vi "Lab Panel V4.84.vi"() -> ()   [LabVIEW 2013] (continued)
            n212 = case shown="True" w255 {
              frame False {
                n213 = local write "Message"("") -> ()
              }
              frame True {
                "Message" <- "NETWORK DIRECTORY NOT FOUND!!!!"
              }
            }
            n214 = property on="Message" class="Str"("Text.TextColor"=u32 16711680) -> ()  [unwired: 2 in, 2 out]
            n215 = property on="Network Directory" class="Path"("Blinking"=w253) -> ()  [unwired: 2 in, 2 out]
            n216 = property on="Message" class="Str"("Blinking"=w253) -> ()  [unwired: 2 in, 2 out]
          }
        }
        frame #10 {
          w261 = FALSE
          n217 = property on="Message" class="Str"("Blinking"=w261) -> ()  [unwired: 2 in, 2 out]
          n218 = property on="Network Directory" class="Path"("Blinking"=w261) -> ()  [unwired: 2 in, 2 out]
          n219 = property on="Tab Control 2" class="TabCtl (strict)"("Value"=0) -> ()  [unwired: 2 in, 2 out]
        }
      }
    }
    frame #2 {
      n220 = node-c288("loop  delay(mS)") -> (w265:T15)  [unwired: 3 in]
      n221 = timed-loop {
        timing: w265 -> [_]
        timing-out: [_] -> w264
        i -> [w287]
        stop <- "stop" stop-if-true
        n222 = node-c288() -> ()  [unwired: 1 in, 1 out]
        n223 = global write "Global display 1.vi" "stop disp"("stop") -> ()
        n224 = local read "SELECT LAB05-2"() -> (w267:T3)
        n225 = local read "SELECT LAB05-1"() -> (w268:T3)
        n226 = local read "SELECT LAB04-2"() -> (w269:T3)
        n227 = local read "SELECT LAB03-1"() -> (w272:T3)
        n228 = local read "SELECT LAB02-2"() -> (w273:T3)
        n229 = local read "SELECT LAB03-2"() -> (w271:T3)
        n230 = local read "SELECT LAB04-1"() -> (w270:T3)
        n231 = local read "SELECT LAB02-1"() -> (w274:T3)
        n232 = local read "TEST LAB01-1"() -> (w276:u16)
        n233 = local read "TEST LAB01-2"() -> (w275:T3)
        n234 = local read "run lab03-2"() -> (w281:bool)
        n235 = local read "run lab04-1"() -> (w280:bool)
        n236 = local read "run lab05-1"() -> (w278:bool)
        n237 = local read "run lab04-2"() -> (w279:bool)
        n238 = local read "run lab05-2"() -> (w277:bool)
        n239 = local read "run lab03-1"() -> (w282:bool)
        n240 = local read "run lab02-2"() -> (w283:bool)
        n241 = local read "run lab02-1"() -> (w284:bool)
        n242 = local read "run lab01-1"() -> (w286:bool)
        n243 = local read "run lab01-2"() -> (w285:bool)
        n244 = stacked-sequence {
          seq-local: [_ w349 _ _ _ _ _ _ _ _ _ _ _ _ _ _ _ _ _ _ _ _] -> [_ _ _ _ _ w2141 _ _ _ _ _ _ _ _ _ _ _ _ _ _ _ _]
          seq-local: [_ w348 _ _ _ _ _ _ _ _ _ _ _ _ _ _ _ _ _ _ _ _] -> [_ _ _ _ _ w2140 _ _ _ _ _ _ _ _ _ _ _ _ _ _ _ _]
          seq-local: [_ w335 _ _ _ _ _ _ _ _ _ _ _ _ _ _ _ _ _ _ _ _] -> [_ _ _ _ _ w2139 _ _ _ _ _ _ _ _ _ _ _ _ _ _ _ _]
          seq-local: [_ w334 _ _ _ _ _ _ _ _ _ _ _ _ _ _ _ _ _ _ _ _] -> [_ _ _ _ _ w2138 _ _ _ _ _ _ _ _ _ _ _ _ _ _ _ _]
          seq-local: [_ w333 _ _ _ _ _ _ _ _ _ _ _ _ _ _ _ _ _ _ _ _] -> [_ _ _ _ _ w2137 _ _ _ _ _ _ _ _ _ _ _ _ _ _ _ _]
          seq-local: [_ w332 _ _ _ _ _ _ _ _ _ _ _ _ _ _ _ _ _ _ _ _] -> [_ _ _ _ _ w2136 _ _ _ _ _ _ _ _ _ _ _ _ _ _ _ _]
          seq-local: [_ w331 _ _ _ _ _ _ _ _ _ _ _ _ _ _ _ _ _ _ _ _] -> [_ _ _ _ _ w2135 _ _ _ _ _ _ _ _ _ _ _ _ _ _ _ _]
          seq-local: [_ w330 _ _ _ _ _ _ _ _ _ _ _ _ _ _ _ _ _ _ _ _] -> [_ _ _ _ _ w2134 _ _ _ _ _ _ _ _ _ _ _ _ _ _ _ _]
          seq-local: [_ w329 _ _ _ _ _ _ _ _ _ _ _ _ _ _ _ _ _ _ _ _] -> [_ _ _ _ _ w2133 _ _ _ _ _ _ _ _ _ _ _ _ _ _ _ _]
          seq-local: [_ w328 _ _ _ _ _ _ _ _ _ _ _ _ _ _ _ _ _ _ _ _] -> [_ _ _ _ _ w2132 _ _ _ _ _ _ _ _ _ _ _ _ _ _ _ _]
          tunnel: w286 -> [_ _ w365 w607 w1731 w2161 w2471 w2718 _ _ _ _ w3122 _ w4056 _ _ w4339 w4642 w4824 _ _]
          tunnel: w285 -> [_ _ w364 w605 w1730 w2160 w2472 w2717 _ _ _ _ w3121 _ w4054 _ _ w4338 w4641 w4822 _ _]
          tunnel: w284 -> [_ _ w363 w603 w1729 w2159 w2470 w2716 _ _ _ _ w3120 _ w4052 _ _ w4337 w4640 w4821 _ _]
          tunnel: w283 -> [_ _ w362 w601 w1728 w2158 w2469 w2715 _ _ _ _ w3119 _ w4050 _ _ w4336 w4639 w4820 _ _]
          tunnel: w282 -> [_ _ w361 w599 w1727 w2157 w2468 w2714 _ _ _ _ w3118 _ w4048 _ _ w4335 w4638 w4819 _ _]
          tunnel: w281 -> [_ _ w360 w597 w1726 w2156 w2467 w2713 _ _ _ _ w3117 _ w4046 _ _ w4334 w4637 w4818 _ _]
          tunnel: w280 -> [_ _ w359 w595 w1725 w2155 w2466 w2712 _ _ _ _ w3116 _ w4044 _ _ w4333 w4636 w4817 _ _]
          tunnel: w279 -> [_ _ w358 w593 w1724 w2154 w2465 w2711 _ _ _ _ w3115 _ w4042 _ _ w4332 w4635 w4816 _ _]
          tunnel: w278 -> [_ _ w357 w591 w1723 w2153 w2464 w2710 _ _ _ _ w3114 _ w4040 _ _ w4331 w4634 w4815 _ _]
          tunnel: w277 -> [_ _ w356 w589 w1722 w2152 w2463 w2709 _ _ _ _ w3113 _ w4038 _ _ w4330 w4633 w4814 _ _]
          tunnel: w276 -> [_ _ _ w606 w1721 w2151 _ _ _ _ _ _ _ _ w4058 _ _ _ _ _ w5168 _]
          tunnel: w275 -> [_ _ _ w604 w1720 w2150 _ _ _ _ _ _ _ _ w4053 _ _ _ _ _ w5167 _]
          tunnel: w274 -> [_ _ _ w602 w1719 w2149 _ _ _ _ _ _ _ _ w4051 _ _ _ _ _ w5166 _]
          tunnel: w273 -> [_ _ _ w600 w1718 w2148 _ _ _ _ _ _ _ _ w4049 _ _ _ _ _ w5165 _]
          tunnel: w272 -> [_ _ _ w598 w1717 w2147 _ _ _ _ _ _ _ _ w4047 _ _ _ _ _ w5164 _]
          tunnel: w271 -> [_ _ _ w596 w1716 w2146 _ _ _ _ _ _ _ _ w4045 _ _ _ _ _ w5163 _]
          tunnel: w270 -> [_ _ _ w594 w1715 w2145 _ _ _ _ _ _ _ _ w4043 _ _ _ _ _ w5162 _]
          tunnel: w269 -> [_ _ _ w592 w1714 w2144 _ _ _ _ _ _ _ _ w4041 _ _ _ _ _ w5161 _]
          tunnel: w268 -> [_ _ _ w590 w1713 w2143 _ _ _ _ _ _ _ _ w4039 _ _ _ _ _ w5160 _]
          tunnel: w267 -> [_ _ _ w588 w1712 w2142 _ _ _ _ _ _ _ _ w4037 _ _ _ _ _ w5159 _]
          frame #0 {
            w291 = FALSE
            w296 = 0.5
            # "set up cycle control"
            n245 = local read "jig cycle"() -> (w295:dbl)
            n246 = Divide(x="JIG ON TIME (S)", y=w296) -> (x/y=→"on loops":dbl)
            n247 = Divide(x="JIG OFF TIME (S)", y=w296) -> (x/y=→"off loops":dbl)
            n248 = Increment(x=w295) -> (x+1=w294:dbl)
            n249 = local write "TEMP"(w291) -> ()
            n250 = local write "AI"(w291) -> ()
            n251 = local write "jig cycle"(w294) -> ()
            n252 = event shown="[1] \"ADMIN\": Value Change" {
              selector: _ -> [_ _]
              dyn-events: _ -> [_ _]
              timeout: 10 -> [_ _]
              event Timeout {
                n253 = event-data() -> ()  [unwired: 1 in, 3 out]
              }
              event "ADMIN": Value Change {
                n254 = event-data() -> ()  [unwired: 1 in, 6 out]
                n255 = stacked-sequence {
                  seq-local: [_ w300 _] -> [_ _ w301]
                  frame #0 {
                    n256 = global write "Global 1.vi" "password"("9999") -> ()
                  }
                  frame #1 {
                    n257 = call "sub vi - password 1.vi"() -> ("RESULT"=w300:bool)  [unwired: 11 in]
                  }
                  frame #2 {
                    w303 = FALSE
                    n258 = property on="Tab Control 2" class="TabCtl (strict)"() -> ("Pages"=w307:refnum<vi>[])  [unwired: 2 in, 2 out]
                    n259 = Select(t=TRUE, s=w301, f=w303) -> (s? t:f=w302:bool)
                    n260 = Index Array(array=w307, index=9) -> (element=w305:refnum<vi>)
                    n261 = property class="Page"(reference=w305, "PageVis"=w302) -> ()  [unwired: 1 in, 2 out]
                    n262 = local write "ADMIN"(w303) -> ()
                  }
                }
              }
            }
          }
          frame #1 {
            w345 = 60.0
            # "convert temperature rise minutes to cycles"
            n263 = local read "SET LAB05-2"() -> (w309:T5)
            n264 = local read "SET LAB05-1"() -> (w311:T5)
            n265 = local read "SET LAB04-2"() -> (w313:T5)
            n266 = local read "SET LAB01-1"() -> (w327:T5)
            n267 = local read "SET LAB01-2"() -> (w325:T5)
            n268 = local read "SET LAB02-2"() -> (w321:T5)
            n269 = local read "SET LAB04-1"() -> (w315:T5)
            n270 = local read "SET LAB03-1"() -> (w319:T5)
            n271 = local read "SET LAB03-2"() -> (w317:T5)
            n272 = local read "SET LAB02-1"() -> (w323:T5)
            n273 = local read "JIG OFF TIME (S)"() -> (w350:dbl)
            n274 = local read "JIG ON TIME (S)"() -> (w351:dbl)
            n275 = Unbundle(w309) -> ("T-RISE mins"=w308:dbl)  [unwired: 4 out]
            n276 = Unbundle(w311) -> ("T-RISE mins"=w310:dbl)  [unwired: 4 out]
            n277 = Unbundle(w327) -> ("T-RISE mins"=w326:dbl)  [unwired: 4 out]
            n278 = Unbundle(w313) -> ("T-RISE mins"=w312:dbl)  [unwired: 4 out]
            n279 = Unbundle(w325) -> ("T-RISE mins"=w324:dbl)  [unwired: 4 out]
            n280 = Unbundle(w323) -> ("T-RISE mins"=w322:dbl)  [unwired: 4 out]
            n281 = Unbundle(w315) -> ("T-RISE mins"=w314:dbl)  [unwired: 4 out]
            n282 = Unbundle(w321) -> ("T-RISE mins"=w320:dbl)  [unwired: 4 out]
            n283 = Unbundle(w317) -> ("T-RISE mins"=w316:dbl)  [unwired: 4 out]
            n284 = Unbundle(w319) -> ("T-RISE mins"=w318:dbl)  [unwired: 4 out]
            n285 = Add(x=w351, y=w350) -> (x+y=w344:dbl)
            n286 = Multiply(x=w345, y=w316) -> (x*y=w340:dbl)
            n287 = Multiply(x=w345, y=w314) -> (x*y=w339:dbl)
            n288 = Multiply(x=w345, y=w312) -> (x*y=w338:dbl)
            n289 = Multiply(x=w345, y=w310) -> (x*y=w337:dbl)
            n290 = Multiply(x=w345, y=w308) -> (x*y=w336:dbl)
            n291 = Multiply(x=w345, y=w324) -> (x*y=w346:dbl)
            n292 = Multiply(x=w345, y=w318) -> (x*y=w341:dbl)
            n293 = Multiply(x=w345, y=w326) -> (x*y=w347:dbl)
            n294 = Multiply(x=w345, y=w322) -> (x*y=w343:dbl)
            n295 = Multiply(x=w345, y=w320) -> (x*y=w342:dbl)
            n296 = Divide(x=w337, y=w344) -> (x/y=w329:dbl)
            n297 = Divide(x=w338, y=w344) -> (x/y=w330:dbl)
            n298 = Divide(x=w339, y=w344) -> (x/y=w331:dbl)
            n299 = Divide(x=w336, y=w344) -> (x/y=w328:dbl)
            n300 = Divide(x=w341, y=w344) -> (x/y=w333:dbl)
            n301 = Divide(x=w347, y=w344) -> (x/y=w349:dbl)
            n302 = Divide(x=w346, y=w344) -> (x/y=w348:dbl)
            n303 = Divide(x=w343, y=w344) -> (x/y=w335:dbl)
            n304 = Divide(x=w342, y=w344) -> (x/y=w334:dbl)
            n305 = Divide(x=w340, y=w344) -> (x/y=w332:dbl)
          }
          frame #2 {
            # "control cycle loops"
            n306 = local read "JIG OFF TIME (S)"() -> (w354:dbl)
            n307 = local read "JIG ON TIME (S)"() -> (w353:dbl)
            n308 = local read "jig cycle"() -> (w367:dbl)
            n309 = local read "on loops"() -> (w369:dbl)
            n310 = local read "off loops"() -> (w368:dbl)
            n311 = Add(x=w354, y=w353) -> (x+y=w352:dbl)
            n312 = Add(x=w369, y=w368) -> (x+y=w355:dbl)
            n313 = Greater Or Equal?(x=w367, y=w355) -> (x >= y?=w366:bool)
            n314 = case shown="True" w366 {
              tunnel: w365 -> [_ w404]
              tunnel: w364 -> [_ w403]
              tunnel: w363 -> [_ w402]
              tunnel: w362 -> [_ w401]
              tunnel: w361 -> [_ w400]
              tunnel: w360 -> [_ w399]
              tunnel: w359 -> [_ w398]
              tunnel: w358 -> [_ w397]
              tunnel: w357 -> [_ w396]
              tunnel: w356 -> [_ w395]
              tunnel: w352 -> [_ w394]
              frame False {
              }
              frame True {
                # "increment cycle value and convert cycles to minutes for temp rise"
                n315 = local read "Panel #"() -> (w371:dbl)
                n316 = local read "JIG RELAY CYCLES"() -> (w393:T7)
                n317 = Increment(x=w371) -> (x+1=w370:dbl)
                n318 = local write "Panel #"(w370) -> ()
                n319 = Unbundle By Name(w393) -> ("LAB01-1"=w391:dbl, "LAB01-2"=w389:dbl, "LAB02-1"=w387:dbl, "LAB02-2"=w385:dbl, "LAB03-1"=w383:dbl, "LAB03-2"=w381:dbl, "LAB04-1"=w379:dbl, "LAB04-2"=w377:dbl, "LAB05-1"=w375:dbl, "LAB05-2"=w373:dbl)
                n320 = stacked-sequence {
                  tunnel: w404 -> [w416 _ _ _ _ _ _ _ _ _]
                  tunnel: w403 -> [_ w433 _ _ _ _ _ _ _ _]
                  tunnel: w402 -> [_ _ w450 _ _ _ _ _ _ _]
                  tunnel: w401 -> [_ _ _ w467 _ _ _ _ _ _]
                  tunnel: w400 -> [_ _ _ _ w484 _ _ _ _ _]
                  tunnel: w399 -> [_ _ _ _ _ w501 _ _ _ _]
                  tunnel: w398 -> [_ _ _ _ _ _ w518 _ _ _]
                  tunnel: w397 -> [_ _ _ _ _ _ _ w535 _ _]
                  tunnel: w396 -> [_ _ _ _ _ _ _ _ w552 _]
                  tunnel: w395 -> [_ _ _ _ _ _ _ _ _ w569]
                  tunnel: w394 -> [w413 w430 w447 w464 w481 w498 w515 w532 w549 w566]
                  tunnel: w391 -> [w407 _ _ _ _ _ _ _ _ _]
                  tunnel: [w406 _ _ _ _ _ _ _ _ _] -> w390
                  tunnel: w389 -> [_ w424 _ _ _ _ _ _ _ _]
                  tunnel: [_ w423 _ _ _ _ _ _ _ _] -> w388
                  tunnel: w387 -> [_ _ w441 _ _ _ _ _ _ _]
                  tunnel: [_ _ w440 _ _ _ _ _ _ _] -> w386
                  tunnel: w385 -> [_ _ _ w458 _ _ _ _ _ _]
                  tunnel: [_ _ _ w457 _ _ _ _ _ _] -> w384
                  tunnel: w383 -> [_ _ _ _ w475 _ _ _ _ _]
                  tunnel: [_ _ _ _ w474 _ _ _ _ _] -> w382
                  tunnel: w381 -> [_ _ _ _ _ w492 _ _ _ _]
                  tunnel: [_ _ _ _ _ w491 _ _ _ _] -> w380
                  tunnel: w379 -> [_ _ _ _ _ _ w509 _ _ _]
                  tunnel: [_ _ _ _ _ _ w508 _ _ _] -> w378
                  tunnel: w377 -> [_ _ _ _ _ _ _ w526 _ _]
                  tunnel: [_ _ _ _ _ _ _ w525 _ _] -> w376
                  tunnel: w375 -> [_ _ _ _ _ _ _ _ w543 _]
                  tunnel: [_ _ _ _ _ _ _ _ w542 _] -> w374
                  tunnel: w373 -> [_ _ _ _ _ _ _ _ _ w560]
                  tunnel: [_ _ _ _ _ _ _ _ _ w559] -> w372
                  frame #0 {
                    n321 = local read "DISP LAB01-1"() -> (w411:T4)
                    n322 = Unbundle(w411) -> ("CYCLE"=w412:dbl)  [unwired: 2 out]
                    n323 = case shown="True" w416 {
                      tunnel: w412 -> [w418 w422]
                      tunnel: [w418 w421] -> w410
                      tunnel: w407 -> [w417 w420]
                      tunnel: [w417 w419] -> w406
                      frame False {
                      }
                      frame True {
                        n324 = Increment(x=w420) -> (x+1=w419:dbl)
                        n325 = Increment(x=w422) -> (x+1=w421:dbl)
                      }
                    }
                    n326 = Multiply(x=w410, y=w413) -> (x*y=w414:dbl)
                    n327 = Divide(x=w414, y=60.0) -> (x/y=w409:dbl)
                    n328 = Bundle(cluster=w411, "CYCLE"=w410, "MINS"=w409) -> (w408:T4)  [unwired: 1 in]
                    n329 = local write "DISP LAB01-1"(w408) -> ()
                  }
                  frame #1 {
                    n330 = local read "DISP LAB01-2"() -> (w428:T4)
                    n331 = Unbundle(w428) -> ("CYCLE"=w429:dbl)  [unwired: 2 out]
                    n332 = case shown="True" w433 {
                      tunnel: w429 -> [w435 w439]
                      tunnel: [w435 w438] -> w426
                      tunnel: w424 -> [w434 w437]
                      tunnel: [w434 w436] -> w423
                      frame False {
                      }
                      frame True {
                        n333 = Increment(x=w437) -> (x+1=w436:dbl)
                        n334 = Increment(x=w439) -> (x+1=w438:dbl)
                      }
                    }
                    n335 = Multiply(x=w426, y=w430) -> (x*y=w431:dbl)
                    n336 = Divide(x=w431, y=60.0) -> (x/y=w425:dbl)
                    n337 = Bundle(cluster=w428, "CYCLE"=w426, "MINS"=w425) -> (w427:T4)  [unwired: 1 in]
                    n338 = local write "DISP LAB01-2"(w427) -> ()
                  }
                  frame #2 {
                    n339 = local read "DISP LAB02-1"() -> (w445:T4)
                    n340 = Unbundle(w445) -> ("CYCLE"=w446:dbl)  [unwired: 2 out]
                    n341 = case shown="True" w450 {
                      tunnel: [w452 w456] -> w443
                      tunnel: w446 -> [w452 w455]
                      tunnel: w441 -> [w451 w454]
                      tunnel: [w451 w453] -> w440
                      frame False {
                      }
                      frame True {
                        n342 = Increment(x=w454) -> (x+1=w453:dbl)
                        n343 = Increment(x=w455) -> (x+1=w456:dbl)
                      }
                    }
                    n344 = Multiply(x=w443, y=w447) -> (x*y=w448:dbl)
                    n345 = Divide(x=w448, y=60.0) -> (x/y=w442:dbl)
                    n346 = Bundle(cluster=w445, "CYCLE"=w443, "MINS"=w442) -> (w444:T4)  [unwired: 1 in]
                    n347 = local write "DISP LAB02-1"(w444) -> ()
                  }
                  frame #3 {
                    n348 = local read "DISP LAB02-2"() -> (w462:T4)
                    n349 = Unbundle(w462) -> ("CYCLE"=w463:dbl)  [unwired: 2 out]
                    n350 = case shown="True" w467 {
                      tunnel: [w469 w473] -> w461
                      tunnel: w463 -> [w469 w472]
                      tunnel: w458 -> [w468 w471]
                      tunnel: [w468 w470] -> w457
                      frame False {
                      }
                      frame True {
                        n351 = Increment(x=w471) -> (x+1=w470:dbl)
                        n352 = Increment(x=w472) -> (x+1=w473:dbl)
                      }
                    }
                    n353 = Multiply(x=w461, y=w464) -> (x*y=w465:dbl)
                    n354 = Divide(x=w465, y=60.0) -> (x/y=w460:dbl)
                    n355 = Bundle(cluster=w462, "CYCLE"=w461, "MINS"=w460) -> (w459:T4)  [unwired: 1 in]
                    n356 = local write "DISP LAB02-2"(w459) -> ()
                  }
                  frame #4 {
                    n357 = local read "DISP LAB03-1"() -> (w479:T4)
                    n358 = Unbundle(w479) -> ("CYCLE"=w480:dbl)  [unwired: 2 out]
                    n359 = case shown="True" w484 {
                      tunnel: [w486 w490] -> w476
                      tunnel: w480 -> [w486 w489]
                      tunnel: w475 -> [w485 w488]
                      tunnel: [w485 w487] -> w474
                      frame False {
                      }
                      frame True {
                        n360 = Increment(x=w488) -> (x+1=w487:dbl)
                        n361 = Increment(x=w489) -> (x+1=w490:dbl)
                      }
                    }
                    n362 = Multiply(x=w476, y=w481) -> (x*y=w482:dbl)
                    n363 = Divide(x=w482, y=60.0) -> (x/y=w477:dbl)
                    n364 = Bundle(cluster=w479, "CYCLE"=w476, "MINS"=w477) -> (w478:T4)  [unwired: 1 in]
                    n365 = local write "DISP LAB03-1"(w478) -> ()
                  }
                  frame #5 {
                    n366 = local read "DISP LAB03-2"() -> (w496:T4)
                    n367 = Unbundle(w496) -> ("CYCLE"=w497:dbl)  [unwired: 2 out]
                    n368 = case shown="True" w501 {
                      tunnel: [w503 w507] -> w495
                      tunnel: w497 -> [w503 w506]
                      tunnel: w492 -> [w502 w505]
                      tunnel: [w502 w504] -> w491
                      frame False {
                      }
                      frame True {
                        n369 = Increment(x=w505) -> (x+1=w504:dbl)
                        n370 = Increment(x=w506) -> (x+1=w507:dbl)
                      }
                    }
                    n371 = Multiply(x=w495, y=w498) -> (x*y=w499:dbl)
                    n372 = Divide(x=w499, y=60.0) -> (x/y=w494:dbl)
                    n373 = Bundle(cluster=w496, "CYCLE"=w495, "MINS"=w494) -> (w493:T4)  [unwired: 1 in]
                    n374 = local write "DISP LAB03-2"(w493) -> ()
                  }
                  frame #6 {
                    n375 = local read "DISP LAB04-1"() -> (w513:T4)
                    n376 = Unbundle(w513) -> ("CYCLE"=w514:dbl)  [unwired: 2 out]
                    n377 = case shown="True" w518 {
                      tunnel: [w520 w524] -> w511
                      tunnel: w514 -> [w520 w523]
                      tunnel: w509 -> [w519 w522]
                      tunnel: [w519 w521] -> w508
                      frame False {
                      }
                      frame True {
                        n378 = Increment(x=w522) -> (x+1=w521:dbl)
                        n379 = Increment(x=w523) -> (x+1=w524:dbl)
                      }
                    }
                    n380 = Multiply(x=w511, y=w515) -> (x*y=w516:dbl)
                    n381 = Divide(x=w516, y=60.0) -> (x/y=w510:dbl)
                    n382 = Bundle(cluster=w513, "CYCLE"=w511, "MINS"=w510) -> (w512:T4)  [unwired: 1 in]
                    n383 = local write "DISP LAB04-1"(w512) -> ()
                  }
                  frame #7 {
                    n384 = local read "DISP LAB04-2"() -> (w530:T4)
                    n385 = Unbundle(w530) -> ("CYCLE"=w531:dbl)  [unwired: 2 out]
                    n386 = case shown="True" w535 {
                      tunnel: [w537 w541] -> w528
                      tunnel: w531 -> [w537 w540]
                      tunnel: w526 -> [w536 w539]
                      tunnel: [w536 w538] -> w525
                      frame False {
                      }
                      frame True {
                        n387 = Increment(x=w539) -> (x+1=w538:dbl)
                        n388 = Increment(x=w540) -> (x+1=w541:dbl)
                      }
                    }
                    n389 = Multiply(x=w528, y=w532) -> (x*y=w534:dbl)
                    n390 = Divide(x=w534, y=60.0) -> (x/y=w527:dbl)
                    n391 = Bundle(cluster=w530, "CYCLE"=w528, "MINS"=w527) -> (w529:T4)  [unwired: 1 in]
                    n392 = local write "DISP LAB04-2"(w529) -> ()
                  }
                  frame #8 {
                    n393 = local read "DISP LAB05-1"() -> (w547:T4)
                    n394 = Unbundle(w547) -> ("CYCLE"=w548:dbl)  [unwired: 2 out]
                    n395 = case shown="True" w552 {
                      tunnel: [w554 w558] -> w545
                      tunnel: w548 -> [w554 w557]
                      tunnel: w543 -> [w553 w556]
                      tunnel: [w553 w555] -> w542
                      frame False {
                      }
                      frame True {
                        n396 = Increment(x=w556) -> (x+1=w555:dbl)
                        n397 = Increment(x=w557) -> (x+1=w558:dbl)
                      }
                    }
                    n398 = Multiply(x=w545, y=w549) -> (x*y=w550:dbl)
                    n399 = Divide(x=w550, y=60.0) -> (x/y=w544:dbl)
                    n400 = Bundle(cluster=w547, "CYCLE"=w545, "MINS"=w544) -> (w546:T4)  [unwired: 1 in]
                    n401 = local write "DISP LAB05-1"(w546) -> ()
                  }
                  frame #9 {
                    n402 = local read "DISP LAB05-2"() -> (w565:T4)
                    n403 = Unbundle(w565) -> ("CYCLE"=w564:dbl)  [unwired: 2 out]
                    n404 = case shown="True" w569 {
                      tunnel: [w571 w575] -> w563
                      tunnel: w564 -> [w571 w574]
                      tunnel: w560 -> [w570 w573]
                      tunnel: [w570 w572] -> w559
                      frame False {
                      }
                      frame True {
                        n405 = Increment(x=w573) -> (x+1=w572:dbl)
                        n406 = Increment(x=w574) -> (x+1=w575:dbl)
                      }
                    }
                    n407 = Multiply(x=w563, y=w566) -> (x*y=w567:dbl)
                    n408 = Divide(x=w567, y=60.0) -> (x/y=w562:dbl)
                    n409 = Bundle(cluster=w565, "CYCLE"=w563, "MINS"=w562) -> (w561:T4)  [unwired: 1 in]
                    n410 = local write "DISP LAB05-2"(w561) -> ()
                  }
                }
                n411 = local write "jig cycle"(0) -> ()
                n412 = Bundle By Name(cluster=w393, "LAB01-1"=w390, "LAB01-2"=w388, "LAB02-1"=w386, "LAB02-2"=w384, "LAB03-1"=w382, "LAB03-2"=w380, "LAB04-1"=w378, "LAB04-2"=w376, "LAB05-1"=w374, "LAB05-2"=w372) -> (w392:T7)
                n413 = local write "JIG RELAY CYCLES"(w392) -> ()
              }
            }
          }
          frame #3 {
            # "START & STOP test RUN switch change, start test if true and stop test if false"
            n414 = Get Date/Time In Seconds() -> (seconds since 1Jan1904=w586:timestamp)
            n415 = local read "C drive data root dir"() -> (w579:path)
            n416 = Format Date/Time String(time format string (%c)="%b\\%a%d", seconds (now)=w586) -> (date/time string=w610:string)  [unwired: 1 in]
            n417 = Format Date/Time String(time format string (%c)="%H%M", seconds (now)=w586) -> (date/time string=w608:string)  [unwired: 1 in]
            n418 = Format Date/Time String(time format string (%c)="LabPanel%Y", seconds (now)=w586) -> (date/time string=w585:string)  [unwired: 1 in]
            n419 = Path To String(path=w579) -> (string=w582:string)
            n420 = global write "Global 1.vi" "C drive root path"(w579) -> ()
            n421 = Concatenate Strings(w582, "\\") -> (w580:string)
            n422 = event shown="[1] \"RUN LAB01-1\": Value Change" {
              selector: _ -> [_ _ _ _ _ _ _ _ _ _ _]
              dyn-events: _ -> [_ _ _ _ _ _ _ _ _ _ _]
              timeout: 10 -> [_ _ _ _ _ _ _ _ _ _ _]
              tunnel: w580 -> [_ w621 w731 w841 w951 w1061 w1171 w1281 w1391 w1501 w1611]
              tunnel: w610 -> [_ w620 w730 w840 w950 w1060 w1170 w1280 w1390 w1500 w1610]
              tunnel: w608 -> [_ w618 w729 w839 w949 w1059 w1169 w1279 w1389 w1499 w1609]
              tunnel: w606 -> [_ w619 _ _ _ _ _ _ _ _ _]
              tunnel: w607 -> [_ _ _ _ _ _ _ _ _ _ _]
              tunnel: w605 -> [_ _ _ _ _ _ _ _ _ _ _]
              tunnel: w604 -> [_ _ w728 _ _ _ _ _ _ _ _]
              tunnel: w603 -> [_ _ _ _ _ _ _ _ _ _ _]
              tunnel: w602 -> [_ _ _ w838 _ _ _ _ _ _ _]
              tunnel: w601 -> [_ _ _ _ _ _ _ _ _ _ _]
              tunnel: w600 -> [_ _ _ _ w948 _ _ _ _ _ _]
              tunnel: w599 -> [_ _ _ _ _ _ _ _ _ _ _]
              tunnel: w598 -> [_ _ _ _ _ w1058 _ _ _ _ _]
              tunnel: w597 -> [_ _ _ _ _ _ _ _ _ _ _]
              tunnel: w596 -> [_ _ _ _ _ _ w1168 _ _ _ _]
              tunnel: w595 -> [_ _ _ _ _ _ _ _ _ _ _]
              tunnel: w594 -> [_ _ _ _ _ _ _ w1278 _ _ _]
              tunnel: w593 -> [_ _ _ _ _ _ _ _ _ _ _]
              tunnel: w592 -> [_ _ _ _ _ _ _ _ w1388 _ _]
              tunnel: w591 -> [_ _ _ _ _ _ _ _ _ _ _]
              tunnel: w590 -> [_ _ _ _ _ _ _ _ _ w1498 _]
              tunnel: w589 -> [_ _ _ _ _ _ _ _ _ _ _]
              tunnel: w588 -> [_ _ _ _ _ _ _ _ _ _ w1608]
              tunnel: w585 -> [_ w617 w727 w837 w947 w1057 w1167 w1277 w1387 w1497 w1607]
              tunnel: [_ w616 w726 w836 w946 w1056 w1166 w1276 w1386 w1496 w1606] -> w583
              tunnel: "RESET CYCLES TO ZERO?" -> [_ w614 w724 w834 w944 w1054 w1164 w1274 w1384 w1494 w1604]
              tunnel: "YES" -> [_ w613 w723 w833 w943 w1053 w1163 w1273 w1383 w1493 w1603]
              tunnel: "NO" -> [_ w612 w722 w832 w942 w1052 w1162 w1272 w1382 w1492 w1602]
              event Timeout {
                n423 = event-data() -> ()  [unwired: 1 in, 3 out]
              }
              event "RUN LAB01-1": Value Change {
                n424 = event-data() -> ("NewVal"=w615:bool)  [unwired: 1 in, 5 out]
                n425 = local write "run lab01-1"(w615) -> ()
                n426 = case shown="True" w615 {
                  tunnel: w621 -> [_ w657]
                  tunnel: w620 -> [_ w656]
                  tunnel: w619 -> [w623 w655]
                  tunnel: w618 -> [_ w654]
                  tunnel: w617 -> [_ w653]
                  tunnel: [w622 w652] -> w616
                  tunnel: w614 -> [_ w651]
                  tunnel: w613 -> [_ w650]
                  tunnel: w612 -> [_ w649]
                  frame False {
                    # "stop test"
                    n427 = stacked-sequence {
                      tunnel: w623 -> [_ w635 _]
                      tunnel: [_ w627 _] -> w622
                      frame #0 {
                        n428 = local read "DISP LAB01-1"() -> (w626:T4)
                        n429 = Bundle(cluster=w626, "STATUS"="STOP") -> (w624:T4)  [unwired: 2 in]
                        n430 = local write "DISP LAB01-1"(w624) -> ()
                      }
                      frame #1 {
                        n431 = local read "DISP LAB01-1"() -> (w634:T4)
                        n432 = Unbundle(w634) -> ("CYCLE"=w632:dbl, "MINS"=w633:dbl)  [unwired: 1 out]
                        n433 = case shown="1" w635 {
                          tunnel: w633 -> [_ _ w642]
                          tunnel: w632 -> [w640 w641 _]
                          tunnel: [w640 w641 w642] -> w631
                          frame 0, Default {
                          }
                          frame 1 {
                          }
                          frame 2 {
                          }
                        }
                        n434 = local read "TDMS LAB01-1"() -> (w639:refnum<k34>)
                        n435 = Build Array("STOPPED") -> (w636:string[])
                        n436 = Build Array(w631) -> (w630:dbl[])
                        n437 = TDMS Write(0:w639, 5:"TEST RESULT", 7:w636, 9:w630) -> (4:w628:refnum<k34>, 15:w629:errorcluster)  [unwired: 2 in, 2 out]
                        n438 = TDMS Close(8:w629, 11:w628) -> (0:w627:errorcluster)  [unwired: 1 out]
                      }
                      frame #2 {
                        n439 = stacked-sequence {
                          tunnel: "LAB01-1" -> [w645 w647]
                          frame #0 {
                            n440 = call "sub vi - defrag tdms v1.vi"("panel id"=w645) -> ("error out"=w644:errorcluster)  [unwired: 10 in]
                            n441 = local write "data file error"(w644) -> ()
                          }
                          frame #1 {
                            n442 = call "Save data file to network drive v2.vi"("panel id"=w647) -> ("network file save error"=w646:errorcluster)  [unwired: 9 in, 1 out]
                            n443 = local write "RESULT LAB01-1"(FALSE) -> ()
                            n444 = local write "data file error"(w646) -> ()
                          }
                        }
                      }
                    }
                  }
                  frame True {
                    # "start new test and create test file"
                    n445 = stacked-sequence {
                      seq-local: [w658 _ _ _ _] -> [_ w679 _ _ _]
                      tunnel: w657 -> [w663 _ _ _ _]
                      tunnel: w656 -> [w659 _ _ _ _]
                      tunnel: w655 -> [w673 _ _ _ _]
                      tunnel: w654 -> [w666 _ _ _ _]
                      tunnel: w653 -> [w661 _ _ _ _]
                      tunnel: [_ w680 _ _ _] -> w652
                      tunnel: w651 -> [_ _ _ w701 _]
                      tunnel: w650 -> [_ _ _ w711 _]
                      tunnel: w649 -> [_ _ _ w710 _]
                      frame #0 {
                        w660 = "\\"
                        n446 = case shown="0, Default" w673 {
                          tunnel: ["L01-1-CHART TEST-" "L01-1-CYCLE TEST-" "L01-1-T-RISE TEST-"] -> w669
                          frame 0, Default {
                          }
                          frame 1 {
                          }
                          frame 2 {
                          }
                        }
                        n447 = local read "SET LAB01-1"() -> (w668:T5)
                        n448 = Unbundle(w668) -> ("DESCRIPTION"=w667:string)  [unwired: 4 out]
                        n449 = Concatenate Strings(w663, "\\", w661, w660, w659, w660) -> (w670:string)
                        n450 = String To Path(string=w670) -> (path=w672:path)
                        n451 = Concatenate Strings(w670, w669, w667, "-", w666, ".tdms") -> (w658:string)
                        n452 = Create Folder(path (use dialog)=w672) -> (error out=w671:errorcluster)  [unwired: 2 in, 2 out]
                        n453 = call <vilib>:"Clear Errors.vi"("error in (no error)"=w671) -> ()  [unwired: 6 in, 1 out]
                        n454 = global write "Global 1.vi" "LAB01-1 FILE"(w658) -> ()
                      }
                      frame #1 {
                        (unwired) FALSE
                        n455 = String To Path(string=w679) -> (path=w677:path)
                        n456 = TDMS Open(6:FALSE, 10:T18."create or replace" ("operation (0:open)"), 11:w677) -> (0:w680:errorcluster, 3:→"TDMS LAB01-1":refnum<k34>)  [unwired: 4 in]
                      }
                      frame #2 {
                        n457 = local read "TDMS LAB01-1"() -> (w699:refnum<k34>)
                        n458 = local read "SET LAB01-1"() -> (w688:T5)
                        n459 = Build Array("Testers Name", "Description", "Set Test Cycles", "T-Rise minutes", "T-Rise Deg C") -> (w689:string[])
                        n460 = Unbundle(w688) -> ("NAME"=w687:string, "DESCRIPTION"=w686:string, "CYCLES"=w685:dbl, "T-RISE mins"=w684:dbl, "T-RISE deg C"=w683:dbl)
                        n461 = Number To Decimal String(number=w685) -> (decimal integer string=w698:string)  [unwired: 1 in]
                        n462 = Number To Decimal String(number=w684) -> (decimal integer string=w697:string)  [unwired: 1 in]
                        n463 = Number To Decimal String(number=w683) -> (decimal integer string=w696:string)  [unwired: 1 in]
                        n464 = Build Array(w687, w686, w698, w697, w696) -> (w695:string[])
                        n465 = TDMS Set Properties(5:w695, 7:w689, 11:w699) -> ()  [unwired: 3 in, 4 out]
                      }
                      frame #3 {
                        n466 = local read "DISP LAB01-1"() -> (w709:T4)
                        n467 = Concatenate Strings("LAB01-1  ", w701) -> (w700:string)
                        n468 = Two Button Dialog(message=w700, 1:w710, 2:w711) -> (T button?=w703:bool)
                        n469 = case shown="True" w703 {
                          tunnel: w709 -> [w714 w715]
                          tunnel: [w714 w715] -> w708
                          tunnel: [w713 w716] -> w707
                          tunnel: [w712 w716] -> w706
                          frame False {
                            n470 = Unbundle(w714) -> ("CYCLE"=w713:dbl, "MINS"=w712:dbl)  [unwired: 1 out]
                          }
                          frame True {
                            w716 = 0.0
                          }
                        }
                        n471 = Bundle(cluster=w708, "CYCLE"=w707, "MINS"=w706, "STATUS"="RUN") -> (w705:T4)
                        n472 = local write "DISP LAB01-1"(w705) -> ()
                      }
                      frame #4 {
                        n473 = local read "SIG LAB01-1"() -> (w719:T2)
                        n474 = local read "TEMP START LAB01-1"() -> (w721:cluster{"TL":dbl, "TN":dbl})
                        n475 = Unbundle(w719) -> ("Tmp Live"=w718:dbl, "Tmp Neut"=w717:dbl)  [unwired: 3 out]
                        n476 = Bundle(cluster=w721, "TL"=w718, "TN"=w717) -> (w720:cluster{"TL":dbl, "TN":dbl})
                        n477 = local write "TEMP START LAB01-1"(w720) -> ()
                      }
                    }
                  }
                }
              }
              event "RUN LAB01-2": Value Change {
                n478 = event-data() -> ("NewVal"=w725:bool)  [unwired: 1 in, 5 out]
                n479 = local write "run lab01-2"(w725) -> ()
                n480 = case shown="True" w725 {
                  tunnel: w731 -> [_ w767]
                  tunnel: w730 -> [_ w766]
                  tunnel: w728 -> [w733 w765]
                  tunnel: w729 -> [_ w764]
                  tunnel: w727 -> [_ w763]
                  tunnel: [w732 w762] -> w726
                  tunnel: w724 -> [_ w761]
                  tunnel: w723 -> [_ w760]
                  tunnel: w722 -> [_ w759]
                  frame False {
                    # "stop test"
                    n481 = stacked-sequence {
                      tunnel: w733 -> [w742 _]
                      tunnel: [w734 _] -> w732
                      frame #0 {
                        n482 = local read "DISP LAB01-2"() -> (w741:T4)
                        n483 = Unbundle(w741) -> ("CYCLE"=w739:dbl, "MINS"=w740:dbl)  [unwired: 1 out]
                        n484 = case shown="\"CHART TEST\", Default" w742 {
                          tunnel: w740 -> [_ _ w749]
                          tunnel: w739 -> [w747 w748 _]
                          tunnel: [w747 w748 w749] -> w738
                          frame "CHART TEST", Default {
                          }
                          frame "CYCLE TEST" {
                          }
                          frame "T-RISE TEST" {
                          }
                        }
                        n485 = local read "TDMS LAB01-2"() -> (w746:refnum<k34>)
                        n486 = Build Array("STOPPED") -> (w743:string[])
                        n487 = Build Array(w738) -> (w737:dbl[])
                        n488 = TDMS Write(0:w746, 5:"TEST RESULT", 7:w743, 9:w737) -> (4:w735:refnum<k34>, 15:w736:errorcluster)  [unwired: 2 in, 2 out]
                        n489 = TDMS Close(8:w736, 11:w735) -> (0:w734:errorcluster)  [unwired: 1 out]
                      }
                      frame #1 {
                        n490 = local read "DISP LAB01-2"() -> (w753:T4)
                        n491 = stacked-sequence {
                          tunnel: "LAB01-2" -> [w755 w757]
                          frame #0 {
                            n492 = call "sub vi - defrag tdms v1.vi"("panel id"=w755) -> ("error out"=w754:errorcluster)  [unwired: 10 in]
                            n493 = local write "data file error"(w754) -> ()
                          }
                          frame #1 {
                            n494 = call "Save data file to network drive v2.vi"("panel id"=w757) -> ("network file save error"=w756:errorcluster)  [unwired: 9 in, 1 out]
                            n495 = local write "RESULT LAB01-2"(FALSE) -> ()
                            n496 = local write "data file error"(w756) -> ()
                          }
                        }
                        n497 = Bundle(cluster=w753, "STATUS"="STOP") -> (w751:T4)  [unwired: 2 in]
                        n498 = local write "DISP LAB01-2"(w751) -> ()
                      }
                    }
                  }
                  frame True {
                    # "start new test and create test file"
                    n499 = stacked-sequence {
                      seq-local: [w768 _ _ _ _] -> [_ w792 _ _ _]
                      tunnel: w767 -> [w773 _ _ _ _]
                      tunnel: w766 -> [w770 _ _ _ _]
                      tunnel: w765 -> [w783 _ _ _ _]
                      tunnel: w764 -> [w776 _ _ _ _]
                      tunnel: w763 -> [w771 _ _ _ _]
                      tunnel: [_ w787 _ _ _] -> w762
                      tunnel: w761 -> [_ _ _ w814 _]
                      tunnel: w760 -> [_ _ _ w813 _]
                      tunnel: w759 -> [_ _ _ w812 _]
                      frame #0 {
                        w769 = "\\"
                        n500 = local read "SET LAB01-2"() -> (w778:T5)
                        n501 = case shown="\"CYCLE TEST\"" w783 {
                          tunnel: ["L01-2-CHART TEST-" "L01-2-CYCLE TEST-" "L01-2-T-RISE TEST-"] -> w779
                          frame "CHART TEST", Default {
                          }
                          frame "CYCLE TEST" {
                          }
                          frame "T-RISE TEST" {
                          }
                        }
                        n502 = Unbundle(w778) -> ("DESCRIPTION"=w777:string)  [unwired: 4 out]
                        n503 = Concatenate Strings(w773, "\\", w771, w769, w770, w769) -> (w780:string)
                        n504 = String To Path(string=w780) -> (path=w782:path)
                        n505 = Concatenate Strings(w780, w779, w777, "-", w776, ".tdms") -> (w768:string)
                        n506 = Create Folder(path (use dialog)=w782) -> (error out=w781:errorcluster)  [unwired: 2 in, 2 out]
                        n507 = global write "Global 1.vi" "LAB01-2 FILE"(w768) -> ()
                        n508 = call <vilib>:"Clear Errors.vi"("error in (no error)"=w781) -> ()  [unwired: 6 in, 1 out]
                      }
                      frame #1 {
                        (unwired) FALSE
                        n509 = String To Path(string=w792) -> (path=w788:path)
                        n510 = TDMS Open(6:FALSE, 10:T18."create or replace" ("operation (0:open)"), 11:w788) -> (0:w787:errorcluster, 3:→"TDMS LAB01-2":refnum<k34>)  [unwired: 4 in]
                      }
                      frame #2 {
                        n511 = local read "SET LAB01-2"() -> (w798:T5)
                        n512 = local read "TDMS LAB01-2"() -> (w809:refnum<k34>)
                        n513 = Build Array("Testers Name", "Description", "Set Test Cycles", "T-Rise minutes", "T-Rise Deg C") -> (w799:string[])
                        n514 = Unbundle(w798) -> ("NAME"=w797:string, "DESCRIPTION"=w796:string, "CYCLES"=w795:dbl, "T-RISE mins"=w794:dbl, "T-RISE deg C"=w793:dbl)
                        n515 = Number To Decimal String(number=w795) -> (decimal integer string=w808:string)  [unwired: 1 in]
                        n516 = Number To Decimal String(number=w794) -> (decimal integer string=w807:string)  [unwired: 1 in]
                        n517 = Number To Decimal String(number=w793) -> (decimal integer string=w806:string)  [unwired: 1 in]
                        n518 = Build Array(w797, w796, w808, w807, w806) -> (w805:string[])
                        n519 = TDMS Set Properties(5:w805, 7:w799, 11:w809) -> ()  [unwired: 3 in, 4 out]
                      }
                      frame #3 {
                        n520 = local read "DISP LAB01-2"() -> (w811:T4)
                        n521 = Concatenate Strings("LAB01-2  ", w814) -> (w815:string)
                        n522 = Two Button Dialog(message=w815, 1:w812, 2:w813) -> (T button?=w817:bool)
                        n523 = case shown="True" w817 {
                          tunnel: w811 -> [w824 w825]
                          tunnel: [w824 w825] -> w821
                          tunnel: [w823 w826] -> w820
                          tunnel: [w822 w826] -> w819
                          frame False {
                            n524 = Unbundle(w824) -> ("CYCLE"=w823:dbl, "MINS"=w822:dbl)  [unwired: 1 out]
                          }
                          frame True {
                            w826 = 0.0
                          }
                        }
                        n525 = Bundle(cluster=w821, "CYCLE"=w820, "MINS"=w819, "STATUS"="RUN") -> (w810:T4)
                        n526 = local write "DISP LAB01-2"(w810) -> ()
                      }
                      frame #4 {
                        n527 = local read "SIG LAB01-2"() -> (w829:T2)
                        n528 = local read "TEMP START LAB01-2"() -> (w831:cluster{"TL":dbl, "TN":dbl})
                        n529 = Unbundle(w829) -> ("Tmp Live"=w828:dbl, "Tmp Neut"=w827:dbl)  [unwired: 3 out]
                        n530 = Bundle(cluster=w831, "TL"=w828, "TN"=w827) -> (w830:cluster{"TL":dbl, "TN":dbl})
                        n531 = local write "TEMP START LAB01-2"(w830) -> ()
                      }
                    }
                  }
                }
              }
              event "RUN LAB02-1": Value Change {
                n532 = event-data() -> ("NewVal"=w835:bool)  [unwired: 1 in, 5 out]
                n533 = local write "run lab02-1"(w835) -> ()
                n534 = case shown="True" w835 {
                  tunnel: w841 -> [_ w877]
                  tunnel: w840 -> [_ w876]
                  tunnel: w838 -> [w843 w875]
                  tunnel: w839 -> [_ w874]
                  tunnel: w837 -> [_ w873]
                  tunnel: [w842 w872] -> w836
                  tunnel: w834 -> [_ w871]
                  tunnel: w833 -> [_ w870]
                  tunnel: w832 -> [_ w869]
                  frame False {
                    # "stop test"
                    n535 = stacked-sequence {
                      tunnel: w843 -> [w852 _]
                      tunnel: [w844 _] -> w842
                      frame #0 {
                        n536 = local read "DISP LAB02-1"() -> (w851:T4)
                        n537 = Unbundle(w851) -> ("CYCLE"=w849:dbl, "MINS"=w850:dbl)  [unwired: 1 out]
                        n538 = case shown="\"CYCLE TEST\"" w852 {
                          tunnel: w850 -> [_ _ w859]
                          tunnel: w849 -> [w857 w858 _]
                          tunnel: [w857 w858 w859] -> w848
                          frame "CHART TEST", Default {
                          }
                          frame "CYCLE TEST" {
                          }
                          frame "T-RISE TEST" {
                          }
                        }
                        n539 = local read "TDMS LAB02-1"() -> (w856:refnum<k34>)
                        n540 = Build Array("STOPPED") -> (w853:string[])
                        n541 = Build Array(w848) -> (w847:dbl[])
                        n542 = TDMS Write(0:w856, 5:"TEST RESULT", 7:w853, 9:w847) -> (4:w845:refnum<k34>, 15:w846:errorcluster)  [unwired: 2 in, 2 out]
                        n543 = TDMS Close(8:w846, 11:w845) -> (0:w844:errorcluster)  [unwired: 1 out]
                      }
                      frame #1 {
                        n544 = local read "DISP LAB02-1"() -> (w863:T4)
                        n545 = stacked-sequence {
                          tunnel: "LAB02-1" -> [w865 w867]
                          frame #0 {
                            n546 = call "sub vi - defrag tdms v1.vi"("panel id"=w865) -> ("error out"=w864:errorcluster)  [unwired: 10 in]
                            n547 = local write "data file error"(w864) -> ()
                          }
                          frame #1 {
                            n548 = local write "RESULT LAB02-1"(FALSE) -> ()
                            n549 = call "Save data file to network drive v2.vi"("panel id"=w867) -> ("network file save error"=w866:errorcluster)  [unwired: 9 in, 1 out]
                            n550 = local write "data file error"(w866) -> ()
                          }
                        }
                        n551 = Bundle(cluster=w863, "STATUS"="STOP") -> (w861:T4)  [unwired: 2 in]
                        n552 = local write "DISP LAB02-1"(w861) -> ()
                      }
                    }
                  }
                  frame True {
                    # "start new test and create test file"
                    n553 = stacked-sequence {
                      seq-local: [w878 _ _ _ _] -> [_ w902 _ _ _]
                      tunnel: w877 -> [w883 _ _ _ _]
                      tunnel: w876 -> [w880 _ _ _ _]
                      tunnel: w875 -> [w893 _ _ _ _]
                      tunnel: w874 -> [w886 _ _ _ _]
                      tunnel: w873 -> [w881 _ _ _ _]
                      tunnel: [_ w897 _ _ _] -> w872
                      tunnel: w871 -> [_ _ _ w923 _]
                      tunnel: w870 -> [_ _ _ w922 _]
                      tunnel: w869 -> [_ _ _ w921 _]
                      frame #0 {
                        w879 = "\\"
                        n554 = local read "SET LAB02-1"() -> (w888:T5)
                        n555 = case shown="\"CYCLE TEST\"" w893 {
                          tunnel: ["L02-1-CHART TEST-" "L02-1-CYCLE TEST-" "L02-1-T-RISE TEST-"] -> w889
                          frame "CHART TEST", Default {
                          }
                          frame "CYCLE TEST" {
                          }
                          frame "T-RISE TEST" {
                          }
                        }
                        n556 = Unbundle(w888) -> ("DESCRIPTION"=w887:string)  [unwired: 4 out]
                        n557 = Concatenate Strings(w883, "\\", w881, w879, w880, w879) -> (w890:string)
                        n558 = String To Path(string=w890) -> (path=w892:path)
                        n559 = Concatenate Strings(w890, w889, w887, "-", w886, ".tdms") -> (w878:string)
                        n560 = Create Folder(path (use dialog)=w892) -> (error out=w891:errorcluster)  [unwired: 2 in, 2 out]
                        n561 = global write "Global 1.vi" "LAB02-1 FILE"(w878) -> ()
                        n562 = call <vilib>:"Clear Errors.vi"("error in (no error)"=w891) -> ()  [unwired: 6 in, 1 out]
                      }
                      frame #1 {
                        (unwired) FALSE
                        n563 = String To Path(string=w902) -> (path=w898:path)
                        n564 = TDMS Open(6:FALSE, 10:T18."create or replace" ("operation (0:open)"), 11:w898) -> (0:w897:errorcluster, 3:→"TDMS LAB02-1":refnum<k34>)  [unwired: 4 in]
                      }
                      frame #2 {
                        n565 = local read "SET LAB02-1"() -> (w908:T5)
                        n566 = local read "TDMS LAB02-1"() -> (w919:refnum<k34>)
